vi "MenuHandler.vi"(5 "tree control":refnum<vi>, 7 "message queue out":T1, 8 "error in (no error)":errorcluster, 9 "parameters":variant, 10 "menu string":string, 11 "NISE_CEF_Node in":refnum<class "NISE_CEF_Node.lvclass">) -> (0 "error out":errorcluster, 2 "Unhandled":bool, 3 "NISE_CEF_Node out":refnum<class "NISE_CEF_Node.lvclass">)   [LabVIEW 2013, in "NISE_CEF_Node.lvclass"]
uses:
  NISE_CEF_Node.lvclass
  <vilib>/NI/AMC/Message Queue.ctl
  <vilib>/NI/AMC/Message.ctl
  <vilib>/NI/Tools/Keyed Array/KeyedArray.ctl
  <vilib>/NI/Tools/Keyed Array/Tools_KeyedArray.lvlib
  <vilib>/NI/AMC/AMC.lvlib
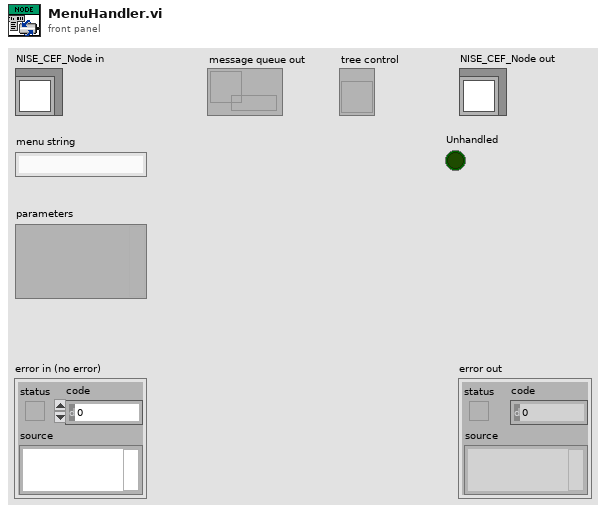
[diagram p1: front panel]
types:
  T1 = typedef "AMC.lvlib/Message Queue.ctl" = refnum<queue>
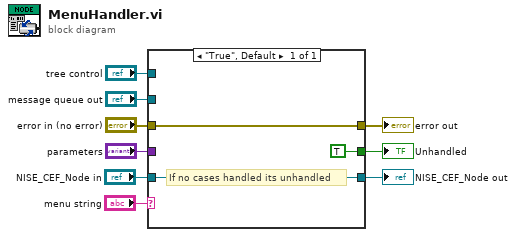
[diagram p0: block diagram]
diagram:
  n1 = case shown="\"True\", Default" "menu string" {
    tunnel: [TRUE ("Unhandled")] -> w8
    tunnel: "parameters" -> [_]
    tunnel: "tree control" -> [_]
    tunnel: "message queue out" -> [_]
    tunnel: "NISE_CEF_Node in" -> [w11]
    tunnel: [w11] -> w3
    tunnel: [w10] -> w1
    tunnel: "error in (no error)" -> [w10]
    frame "True", Default {
      # "If no cases handled its unhandled"
    }
  }
  "error out" <- w1
  "NISE_CEF_Node out" <- w3
  "Unhandled" <- w8
